vi "Add All Projects.vi"(8 "error in (no error)":errorcluster, 9 "Folder":path, 10 "GPack.lvlib:PackageAbstract.lvclass in":refnum<class "PackageAbstract.lvclass">) -> (0 "error out":errorcluster, 2 "GPack.lvlib:PackageAbstract.lvclass out":refnum<class "PackageAbstract.lvclass">)   [LabVIEW 2020, in "GPackTools.lvlib" / "GPackCLI.lvclass"]
uses:
  GPackCLI.lvclass
  GPack/PackageAbstract/PackageAbstract.lvclass
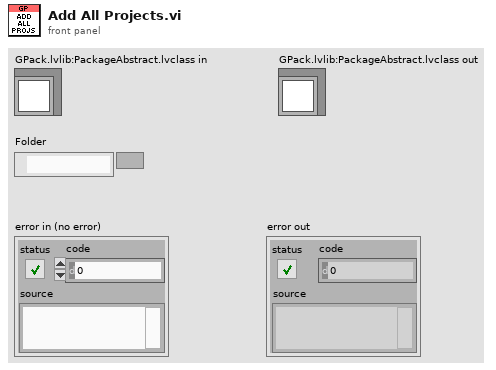
[diagram p1: front panel]
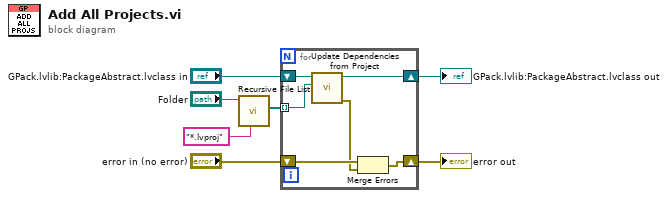
[diagram p0: block diagram]
diagram:
  n1 = call <vilib>:"Recursive File List.vi"("pattern"="*.lvproj", "Folder Path"="Folder") -> ("All Files in Dir"=w5:path[])  [unwired: 5 in, 4 out]
  n2 = for {
    tunnel: w5 -> [w12] mode=indexing
    shift-right: [w8] -> w1
    shift-left: "error in (no error)" -> [w10]
    shift-right: [w11] -> w2
    shift-left: "GPack.lvlib:PackageAbstract.lvclass in" -> [w13]
    n3 = call "Update Dependencies from Project.vi"("lvproj Path"=w12, "PackageAbstract in"=w13) -> ("error out"=w9:errorcluster, "PackageAbstract out"=w11:refnum<class "PackageAbstract.lvclass">)  [unwired: 8 in]
    n4 = Merge Errors(w10, w9) -> (w8:errorcluster)
  }
  "GPack.lvlib:PackageAbstract.lvclass out" <- w2
  "error out" <- w1
